vi "Disable or enable Menu Items.vi"(7 "enabled":bool=TRUE, 8 "error in (no error)":errorcluster, 10 "Item Tags":string[](array[string]), 11 "menu reference":refnum<k9>) -> (0 "error out":errorcluster)   [LabVIEW 2013]
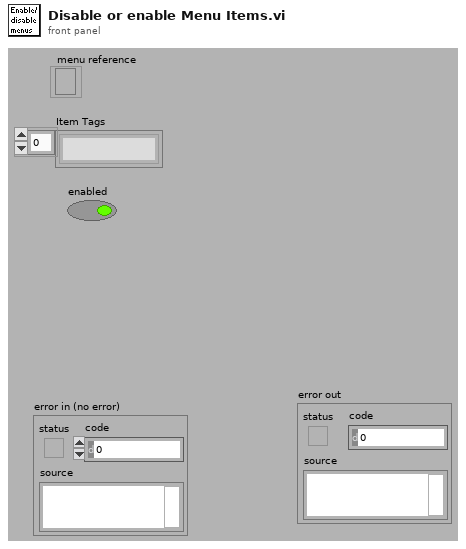
[diagram p1: front panel]
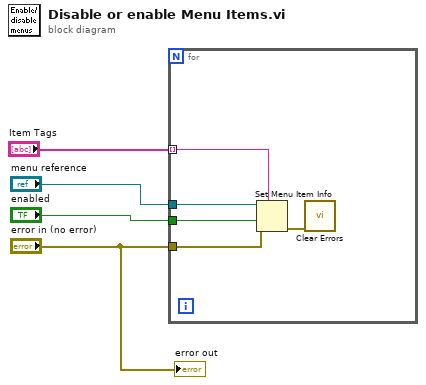
[diagram p0: block diagram]
diagram:
  n1 = for {
    tunnel: "menu reference" -> [w9]
    tunnel: "error in (no error)" -> [w8]
    tunnel: "enabled" -> [w7]
    tunnel: "Item Tags" -> [w5] mode=indexing
    n2 = Set Menu Item Info(7:w5, 8:w8, 9:w7, 11:w9) -> (0:w6:errorcluster)  [unwired: 4 out]
    n3 = call <vilib>:"Clear Errors.vi"("error in (no error)"=w6) -> ()  [unwired: 7 out]
  }
  "error out" <- "error in (no error)"
